vi "ColorCreator.vi"(1 "Reflectance values":dbl[](array[numeric])) -> (0 "Spectrum":dbl[](array[numeric]) format="%_6g")   [LabVIEW 2013]
uses:
  <vilib>/Utility/file.llb/Write To Spreadsheet File (DBL).vi
  <vilib>/gmath/NI_Gmath.lvlib
panel:
  in  "?":bool
  in  "780nm":dbl(slide)=0.001 min=0.001 max=0.99 scale=0.0..1.0 scale format="%1.3f"
  in  "650nm":dbl(slide)=0.001 min=0.001 max=0.99 scale=0.0..1.0 scale format="%1.3f"
  in  "700nm":dbl(slide)=0.001 min=0.001 max=0.99 scale=0.0..1.0 scale format="%1.3f"
  in  "575nm":dbl(slide)=0.001 min=0.001 max=0.99 scale=0.0..1.0 scale format="%1.3f"
  in  "550nm":dbl(slide)=0.001 min=0.001 max=0.99 scale=0.0..1.0 scale format="%1.3f"
  in  "525nm":dbl(slide)=0.001 min=0.001 max=0.99 scale=0.0..1.0 scale format="%1.3f"
  in  "500nm":dbl(slide)=0.001 min=0.001 max=0.99 scale=0.0..1.0 scale format="%1.3f"
  in  "600nm":dbl(slide)=0.001 min=0.001 max=0.99 scale=0.0..1.0 scale format="%1.3f"
  in  "450nm":dbl(slide)=0.001 min=0.001 max=0.99 scale=0.0..1.0 scale format="%1.3f"
  in  "380nm":dbl(slide)=0.001 min=0.001 max=0.99 scale=0.0..1.0 scale format="%1.3f"
  out "XY Graph":cluster{i32[], "yi":dbl[]}(graph)
  in  "Color name":string
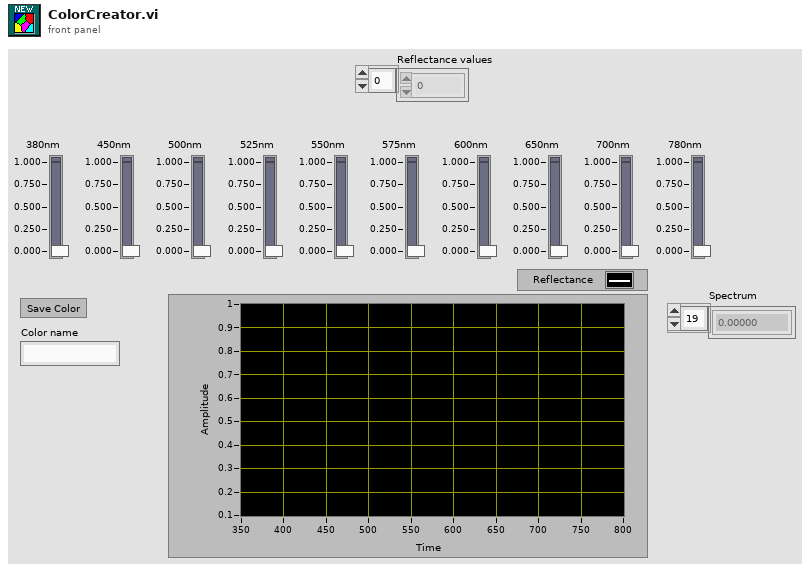
[diagram p1: front panel]
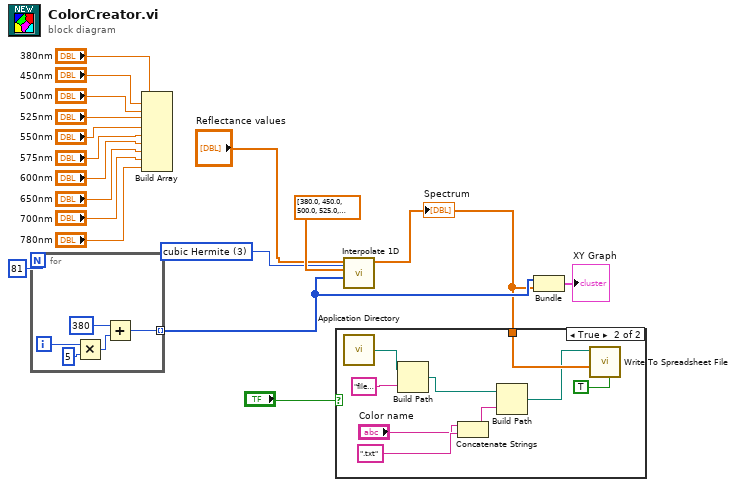
[diagram p0: block diagram]
diagram:
  w3 = 3 items=["nearest", "linear", "spline", "cubic Hermite", "Lagrange"] ("method")
  n1 = for {
    N: 81 -> [_]
    tunnel: [w19] -> w16 mode=indexing
    i -> [w23]
    n2 = Multiply(x=w23, y=5) -> (x*y=w21:i32)
    n3 = Add(x=380, y=w21) -> (x+y=w19:i32)
  }
  n4 = Build Array("380nm", "450nm", "500nm", "525nm", "550nm", "575nm", "600nm", "650nm", "700nm", "780nm") -> ()  [unwired: 1 out]
  n5 = call <vilib>:"Interpolate 1D.vi"("method"=w3, "xi"=w16, "X"=dbl[] [380.0, 450.0, 500.0, 525.0, 550.0, 575.0, 600.0, 650.0, 700.0, 780.0] ("Y"), "Y"="Reflectance values") -> ("yi"=w15:dbl[])  [unwired: 5 in, 2 out]
  "Spectrum" <- w15
  n6 = case shown="True" "?" {
    tunnel: w15 -> [_ w30]
    frame False {
    }
    frame True {
      n7 = call <vilib>:"Application Directory.vi"() -> ("Application Directory"=w28:path)
      n8 = Build Path(base path=w28, name or relative path="files\\colors\\") -> (appended path=w26:path)
      n9 = Concatenate Strings("Color name", ".txt" ("string")) -> (w25:string)
      n10 = Build Path(base path=w26, name or relative path=w25) -> (appended path=w24:path)
      n11 = call-poly <vilib>:"Write To Spreadsheet File.vi"("transpose? (no:F)"=TRUE, "1D data"=w30, "file path (dialog if empty)"=w24) -> ()  [unwired: 5 in, 1 out]
    }
  }
  n12 = Bundle(w16, "yi"=w15) -> (→"XY Graph":cluster{i32[], "yi":dbl[]})  [unwired: 1 in]
